vi "goToBackBall.vi"(6 "target":dbl[](array[numeric]), 8 "error in (no error)":errorcluster, 9 "Ball":refnum<class "Ball.lvclass">, 10 "Robot in":refnum<class "Robot.lvclass">, 11 "KickToSkill in":refnum<class "KickToSkill.lvclass">) -> (0 "error out":errorcluster, 1 "robotKickState":T1, 2 "Robot out":refnum<class "Robot.lvclass">, 3 "KickToSkill out":refnum<class "KickToSkill.lvclass">)   [LabVIEW 2020, in "KickToSkill.lvclass"]
uses:
  KickToSkill.lvclass
  Ball_class/Ball.lvclass
  C:/Users/victo/Desktop/IME/RoboIME/SSL_AI/Object_class/Object.lvclass
  Robot_class/Robot.lvclass
  Robot_class/robotKickToStates.ctl
  Object_class/Object.lvclass/Object.ctl
  Robot_class/Robot.lvclass/Robot.ctl
  <vilib>/Analysis/baseanly.llb/Unit Vector (DBL).vi
  <vilib>/Analysis/_algsub.llb/Real Vector Norm.vi
  <vilib>/Analysis/coordinate.llb/Wrap Angle (scalar).vi
  Robot_class/Read orientation.vi
  Object_class/Read position(x,y).vi
  Robot_class/Write dest_x.vi
  Robot_class/Write dest_y.vi
  Robot_class/Write dest_orientation.vi
  <vilib>/Analysis/NI_AALBase.lvlib
  Utilities_class/Utilities.lvclass
  <vilib>/Analysis/NI_AAL_Angle.lvlib
  <vilib>/Analysis/NI_AALPro.lvlib
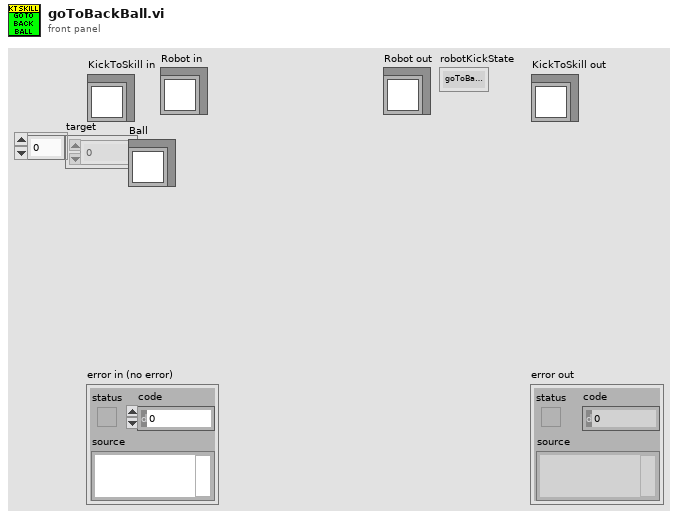
[diagram p1: front panel]
types:
  T1 = typedef "robotKickToStates.ctl" = enum16{"goToBackBall", "none", "andar", "girar", "chutar"}
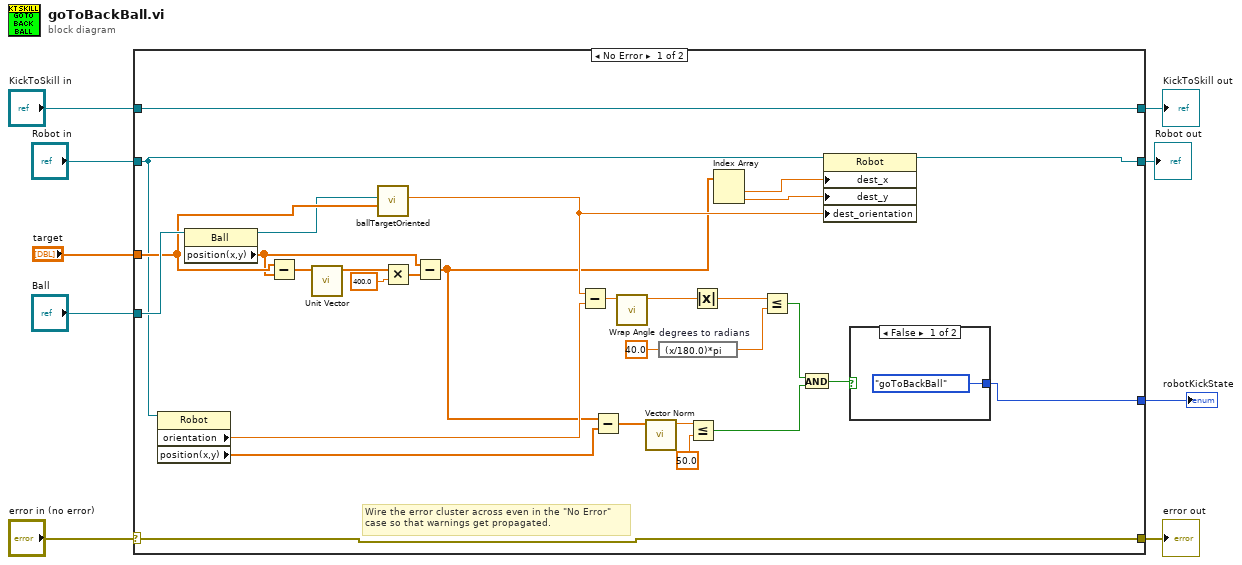
[diagram p0: block diagram]
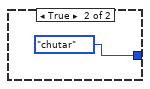
[diagram p2: hidden frame]
diagram:
  n1 = case shown="No Error" "error in (no error)" {
    selector: "error in (no error)" -> [w38 w43]
    tunnel: [w38 w43] -> w8
    tunnel: [w39 w42] -> w6
    tunnel: "KickToSkill in" -> [w39 w42]
    tunnel: "target" -> [w31 _]
    tunnel: "Ball" -> [w37 _]
    tunnel: "Robot in" -> [w28 _]
    tunnel: [w29 _] -> w2
    tunnel: [w10 _] -> w1
    frame No Error {
      # "Wire the error cluster across even in the \"No Error\"\ncase so that warnings get propagated."
      n2 = property class="Robot"(reference=w28) -> ("orientation"=w24:dbl, "position(x,y)"=w18:dbl[])  [unwired: 1 in, 2 out]
      n3 = property class="Ball"(reference=w37) -> (reference out=w30:refnum<class "Ball.lvclass">, "position(x,y)"=w27:dbl[])  [unwired: 1 in, 1 out]
      n4 = Subtract(x=w31, y=w27) -> (x-y=w36:dbl[])
      n5 = call-poly <vilib>:"Unit Vector.vi"("Input Vector"=w36) -> ("Unit Vector"=w35:dbl[])  [unwired: 8 in, 2 out]
      n6 = call "ballTargetOriented.vi"("Target"=w31, "Ball"=w30) -> ("Orientation"=w25:dbl)  [unwired: 7 in, 2 out]
      n7 = Multiply(x=w35, y=400.0) -> (x*y=w34:dbl[])
      n8 = Subtract(x=w27, y=w34) -> (x-y=w17:dbl[])
      n9 = Subtract(x=w25, y=w24) -> (x-y=w23:dbl)
      n10 = Subtract(x=w17, y=w18) -> (x-y=w16:dbl[])
      n11 = call-poly <vilib>:"Wrap Angle.vi"("angle in"=w23) -> ("angle out"=w22:dbl)  [unwired: 9 in, 1 out]
      n12 = call-poly <vilib>:"Vector Norm.vi"("Input Vector"=w16) -> ("norm"=w15:dbl)  [unwired: 9 in, 1 out]
      n13 = expression code="(x/180.0)*pi" "degrees to radians"(40.0) -> (w20:dbl)
      n14 = Less Or Equal?(x=w15, y=50.0) -> (x <= y?=w12:bool)
      n15 = Absolute Value(x=w22) -> (abs(x)=w21:dbl)
      n16 = Index Array(array=w17) -> (element #1=w33:dbl, element #2=w32:dbl)  [unwired: 2 in]
      n17 = Less Or Equal?(x=w21, y=w20) -> (x <= y?=w13:bool)
      n18 = And(x=w13, y=w12) -> (x .and. y?=w11:bool)
      n19 = property class="Robot"(reference=w28, "dest_x"=w33, "dest_y"=w32, "dest_orientation"=w25) -> (reference out=w29:refnum<class "Robot.lvclass">)  [unwired: 1 in, 1 out]
      n20 = case shown="False" w11 {
        tunnel: [robotKickToStates."goToBackBall" ("robotKickState") robotKickToStates."chutar" ("t")] -> w10
        frame False {
        }
        frame True {
        }
      }
    }
    frame Error {
    }
  }
  "error out" <- w8
  "KickToSkill out" <- w6
  "Robot out" <- w2
  "robotKickState" <- w1
